vi "Close 3D-ODE.vi"(8 "error in (no error)":errorcluster, 11 "ODESimulator_Base_Conveyor in":refnum<class "ODESimulator_Base_Conveyor.lvclass">) -> (0 "error out":errorcluster, 3 "ODESimulator_Base_Conveyor out":refnum<class "ODESimulator_Base_Conveyor.lvclass">)   [LabVIEW 2017, in "NI_Robotics_Simulator.lvlib" / "ODESimulator_Base_Conveyor.lvclass"]
uses:
  <vilib>/robotics/Simulator/Robot Factory/Conveyor/Base/ODESimulator_Base_Conveyor.lvclass
  <vilib>/robotics/Simulator/Robot Factory/Conveyor/Base/ODESimulator_Base_Conveyor.lvclass/ODESimulator_Base_Conveyor.ctl
  <vilib>/robotics/Simulator/LVODE/Close Reference (Conveyor).vi
  <vilib>/robotics/Simulator/3D-Physics/Base/3D_Physics_Base.lvclass
  <vilib>/robotics/Simulator/NI_Robotics_Simulator.lvlib
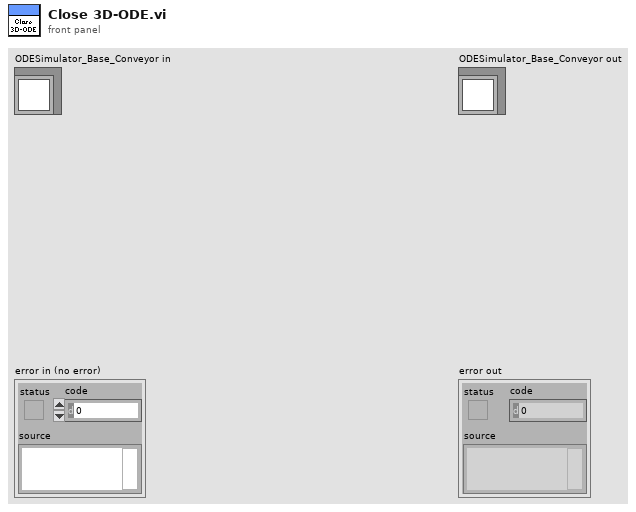
[diagram p1: front panel]
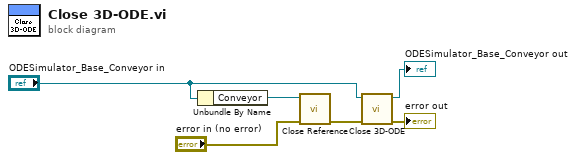
[diagram p0: block diagram]
diagram:
  n1 = Unbundle By Name("ODESimulator_Base_Conveyor in") -> ("Conveyor"=w4:refnum<k20>)
  n2 = call-poly <vilib>:"Close Reference.vi"("error in (no error)"="error in (no error)", "Conveyor"=w4) -> ("error out"=w2:errorcluster)  [unwired: 9 in]
  n3 = call-parent "Close 3D-ODE.vi"("error in (no error)"=w2, "3D_Physics_Base in"="ODESimulator_Base_Conveyor in") -> ("error out"=→"error out":errorcluster, "3D_Physics_Base out"=→"ODESimulator_Base_Conveyor out":refnum<class "ODESimulator_Base_Conveyor.lvclass">)  [unwired: 8 in]
